vi "FeedBackNodeWithOutsideInitializer.vi"() -> ()   [LabVIEW 2019]
panel:
  out "Factorial":u16
  in  "Number":u16
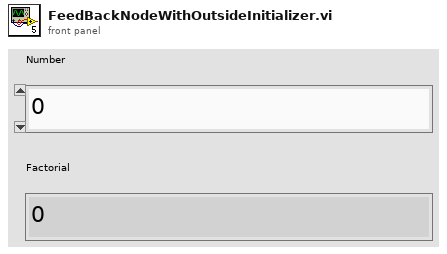
[diagram p1: front panel]
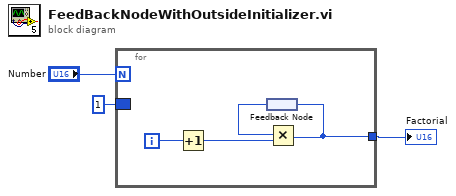
[diagram p0: block diagram]
diagram:
  n1 = for {
    N: "Number" -> [_]
    tunnel: [w4] -> w2
    border: 1 -> [_]
    i -> [w7]
    n2 = Increment(x=w7) -> (x+1=w6:i32)
    n3 = feedback #1() -> (w5:i32)
    n4 = Multiply(x=w5, y=w6) -> (x*y=w4:i32)
    n5 = feedback-in #1(w4) -> ()
  }
  "Factorial" <- w2
